vi "DetectFallingEdge.vi"(10 "Boolean":bool) -> (2 "DetectedEdge":bool)   [LabVIEW 2013]
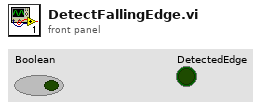
[diagram p1: front panel]
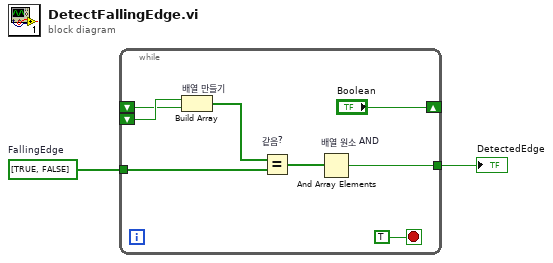
[diagram p0: block diagram]
diagram:
  w1 = bool[] [TRUE, FALSE]  # FallingEdge
  n1 = while {
    shift-right: ["Boolean"] -> _
    shift-left: _ -> [w3]
    tunnel: w1 -> [w7]
    shift-left: _ -> [w4]
    tunnel: [w5] -> w2
    stop <- TRUE stop-if-true
    n2 = Build Array "배열 만들기"(w4, w3) -> (w8:bool[])
    n3 = Equal? "같음?"(x=w8, y=w7) -> (x = y?=w6:bool[])
    n4 = And Array Elements "배열 원소 AND"(Boolean array=w6) -> (logical AND=w5:bool)
  }
  "DetectedEdge" <- w2
